vi "TestBufferProperties.vi"() -> ()   [LabVIEW 2017]
uses:
  kernel32.dll
panel:
  out "error out":errorcluster
  out "Latency after  processing":dbl(graph)
  out "Latency before processing":dbl(graph)
  out "Buffer length (samp)":dbl(graph)
  out "Time b/w buffers (samp)":dbl(graph)
  in  "TTL port":u16=5557
  in  "Stop Button":bool
  in  "TTL channel":u16=1 min=1 max=8
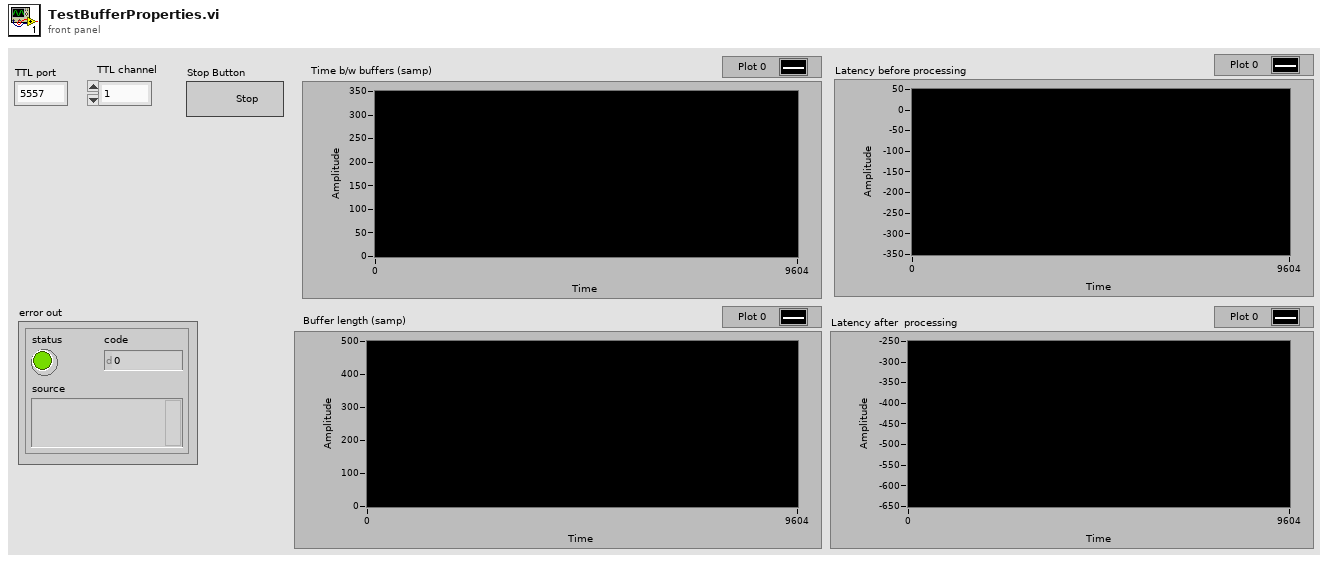
[diagram p1: front panel]
types:
  T1 = enum16{"big-endian, network order", "native, host order", "little-endian"}
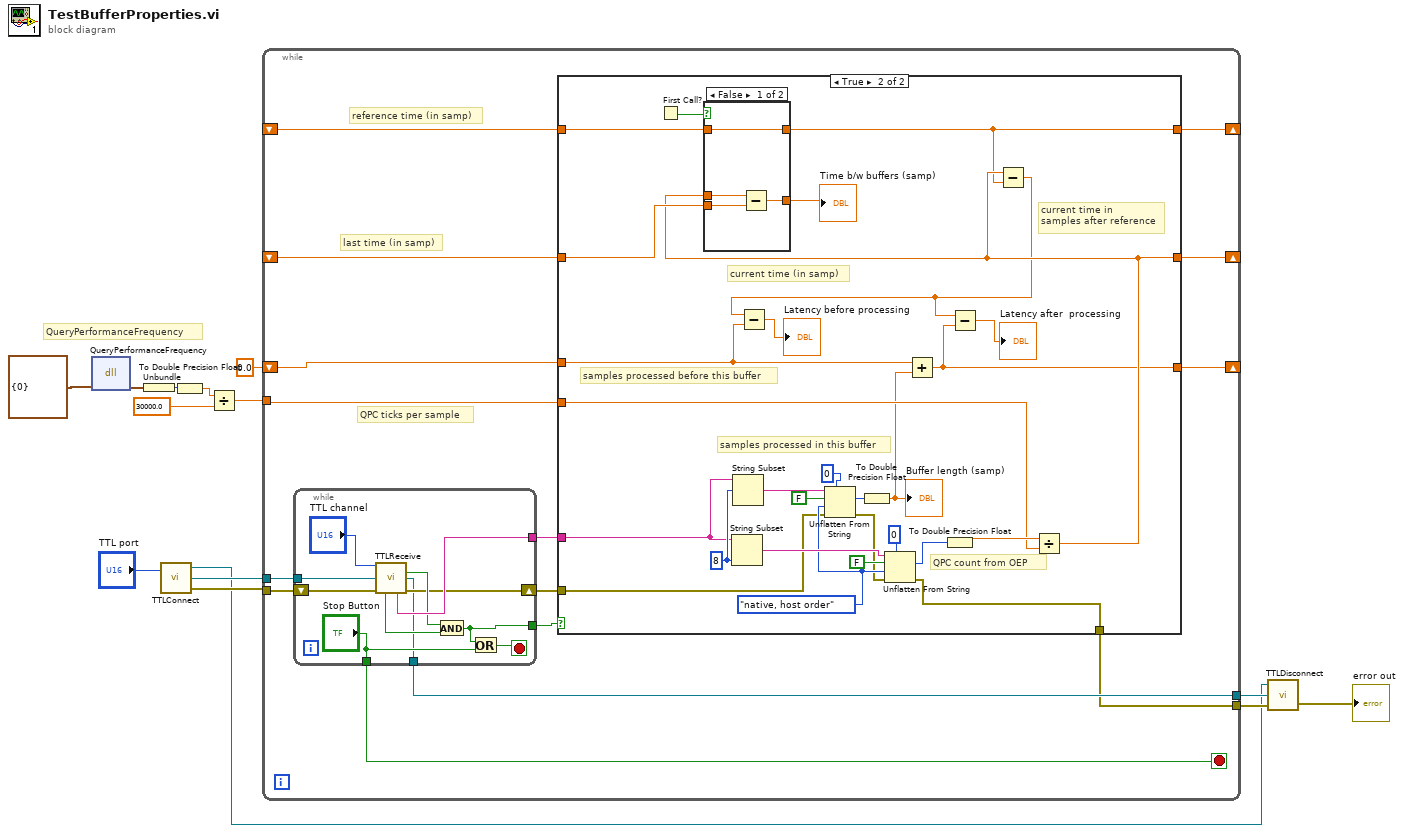
[diagram p0: block diagram]
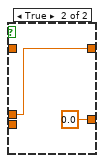
[diagram p3: hidden frame]
diagram:
  # "QueryPerformanceFrequency"
  n1 = dll-call lib="kernel32.dll" fn="QueryPerformanceFrequency"("lpFrequency"=cluster{i64} {0}) -> ("lpFrequency"=w13:cluster{i64})  [unwired: 4 in, 2 out]
  n2 = Unbundle(w13) -> (w12:i64)
  n3 = call "TTLConnect.vi"("port"="TTL port") -> ("context out"=w1:refnum<class "zmq_context.lvclass">, "socket out"=w6:refnum<class "zmq_socket.lvclass">, "error out"=w5:errorcluster)  [unwired: 1 in]
  n4 = To Double Precision Float(number=w12) -> (double precision float=w10:dbl)
  n5 = Divide(x=w10, y=30000.0) -> (x/y=w8:dbl)
  n6 = while {
    tunnel: w6 -> [w19]
    tunnel: w5 -> [w20]
    tunnel: w8 -> [w28]
    shift-right: [w26] -> _
    shift-left: _ -> [w27]
    shift-right: [w25] -> _
    shift-left: _ -> [w24]
    shift-right: [w23] -> _
    shift-left: 0.0 -> [w22]
    tunnel: [w16] -> w3
    tunnel: [w15] -> w2
    stop <- w17 stop-if-true
    # "last time (in samp)"
    # "reference time (in samp)"
    # "QPC ticks per sample"
    n7 = while {
      tunnel: [w40] -> w29
      tunnel: [w32] -> w21
      tunnel: w19 -> [w35]
      shift-right: [w34] -> w18
      shift-left: w20 -> [w36]
      tunnel: ["Stop Button"] -> w17
      tunnel: [w30] -> w16
      stop <- w33 stop-if-true
      n8 = call "TTLReceive.vi"("channel"="TTL channel", "socket in"=w35, "error in"=w36) -> ("new TTL"=w37:bool, "socket out"=w30:refnum<class "zmq_socket.lvclass">, "event on"=w38:bool, "metadata"=w40:string, "error out"=w34:errorcluster)  [unwired: 6 in, 2 out]
      n9 = And(x=w37, y=w38) -> (x .and. y?=w32:bool)
      n10 = Or(x=w32, y="Stop Button") -> (x .or. y?=w33:bool)
    }
    n11 = case shown="True" w21 {
      tunnel: w29 -> [_ w67]
      tunnel: w28 -> [_ w60]
      tunnel: w27 -> [w44 w59]
      tunnel: [w44 w54] -> w26
      tunnel: [w43 w53] -> w25
      tunnel: w24 -> [w43 w56]
      tunnel: [w42 w49] -> w23
      tunnel: w22 -> [w42 w51]
      tunnel: w18 -> [w41 w47]
      tunnel: [w41 w46] -> w15
      frame False {
      }
      frame True {
        w68 = 8 ("length (rest)")
        w64 = T1."native, host order" ("byte order (0:big-endian, network order)")
        # "samples processed in this buffer"
        # "current time in\nsamples after reference"
        # "samples processed before this buffer"
        # "current time (in samp)"
        # "QPC count from OEP"
        n12 = First Call?() -> (First Call?: T/F=w58:bool)
        n13 = String Subset(string=w67, length (rest)=w68) -> (substring=w69:string)  [unwired: 1 in]
        n14 = String Subset(string=w67, offset (0)=w68) -> (substring=w65:string)  [unwired: 1 in]
        n15 = Unflatten From String(type=0, binary string=w65, data includes array or string size? (T)=FALSE, byte order (0:big-endian, network order)=w64, error in (no error)=w47) -> (value=w57:i32, error out=w63:errorcluster)  [unwired: 1 out]
        n16 = To Double Precision Float(number=w57) -> (double precision float=w55:dbl)
        "Buffer length (samp)" <- w55
        n17 = Unflatten From String(type=i64 0, binary string=w69, data includes array or string size? (T)=FALSE, byte order (0:big-endian, network order)=w64, error in (no error)=w63) -> (value=w70:i64, error out=w46:errorcluster)  [unwired: 1 out]
        n18 = Add(x=w51, y=w55) -> (x+y=w49:dbl)
        n19 = To Double Precision Float(number=w70) -> (double precision float=w61:dbl)
        n20 = Divide(x=w61, y=w60) -> (x/y=w54:dbl)
        n21 = case shown="False" w58 {
          tunnel: w59 -> [w76 _]
          tunnel: w54 -> [w74 w78]
          tunnel: [w75 w78] -> w53
          tunnel: w56 -> [w75 _]
          tunnel: [w73 0.0] -> w45
          frame False {
            n22 = Subtract(x=w74, y=w76) -> (x-y=w73:dbl)
          }
          frame True {
          }
        }
        "Time b/w buffers (samp)" <- w45
        n23 = Subtract(x=w54, y=w53) -> (x-y=w52:dbl)
        n24 = Subtract(x=w52, y=w51) -> (x-y=→"Latency before processing":dbl)
        n25 = Subtract(x=w52, y=w49) -> (x-y=→"Latency after  processing":dbl)
      }
    }
  }
  n26 = call "TTLDisconnect.vi"("error in"=w2, "socket in"=w3, "context in"=w1) -> ("error out"=→"error out":errorcluster)  [unwired: 1 in]
